vi "DrawEllipse.vi"() -> ()   [LabVIEW 2022 SP3]
uses:
  System.Windows.Forms
  System.Drawing
panel:
  in  "Numeric":dbl
  in  "stop":bool
  in  "PictureBox":refnum<k24>(container)
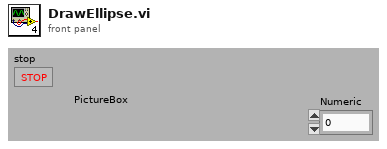
[diagram p1: front panel]
types:
  T1 = cluster{"Event Common Data":cluster{"Event Source":i32, "Event Type":u32, "Time Stamp":u32}, "Control Ref":refnum<k24>, "Event Data":cluster{"sender":refnum<k24>, "e":refnum<k24>}}
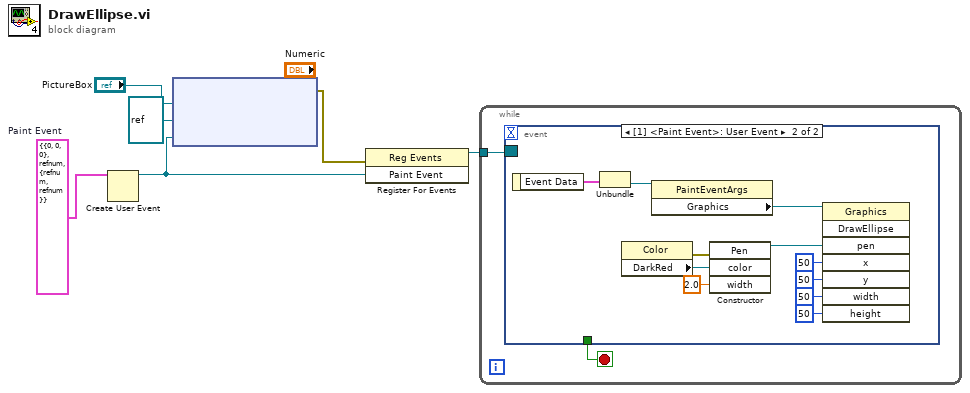
[diagram p0: block diagram]
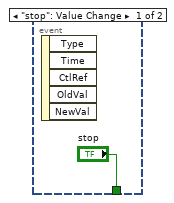
[diagram p2: hidden frame]
diagram:
  w2 = T1 {"Event Common Data"={"Event Source"=0, "Event Type"=0, "Time Stamp"=0}, "Control Ref"=refnum, "Event Data"={"sender"=refnum, "e"=refnum}}  # Paint Event
  n1 = Create User Event(user event datatype=w2) -> (user event=w6:refnum<user-event>)  [unwired: 1 in, 1 out]
  n2 = node("PictureBox", refnum<vi> refnum ("VI Ref"), w6) -> (w3:errorcluster)  [unwired: 2 in, 1 out]
  n3 = register-events(error in=w3, w6) -> (reference out=w5:refnum<event-registration>)  [unwired: 1 in, 1 out]
  n4 = while {
    tunnel: w5 -> [w8]
    stop <- w7 stop-if-true
    n5 = event shown="[1] <Paint Event>: User Event" {
      selector: w8 -> [_ _]
      dyn-events: _ -> [_ _]
      timeout: _ -> [_ _]
      tunnel: ["stop" _] -> w7
      event "stop": Value Change {
        n6 = event-data() -> ()  [unwired: 1 in, 5 out]
      }
      event User Event {
        n7 = event-data() -> ("Event Data"=w20:cluster{"sender":refnum<k24>, "e":refnum<k24>})  [unwired: 1 in]
        n8 = Unbundle(w20) -> ("e"=w19:refnum<k24>)  [unwired: 1 out]
        n9 = property class="Color"() -> (error out=w18:errorcluster, "DarkRed"=w17:refnum<k24>)  [unwired: 2 in, 1 out]
        n10 = property class="PaintEventArgs"(reference=w19) -> ("Graphics"=w10:refnum<k24>)  [unwired: 1 in, 2 out]
        n11 = constructor class="Pen"(error in=w18, "color"=w17, "width"=sgl 2.0) -> (reference out=w11:refnum<k24>)  [unwired: 2 in, 4 out]
        n12 = invoke class="Graphics" method="DrawEllipse"(reference=w10, "pen"=w11, "x"=50, "y"=50, "width"=50, "height"=50) -> ()  [unwired: 2 in, 8 out]
      }
    }
  }
